vi "readU16.vi"(8 "error in (no error)":errorcluster, 11 "ModbusBuffer in":refnum<class "ModbusBuffer.lvclass">) -> (0 "error out":errorcluster, 2 "Output":u16, 3 "ModbusBuffer out":refnum<class "ModbusBuffer.lvclass">)   [LabVIEW 2016, in "RTModbus.lvlib" / "ModbusBuffer.lvclass"]
uses:
  ModbusBuffer.lvclass
  ModbusBuffer.lvclass/ModbusBuffer.ctl
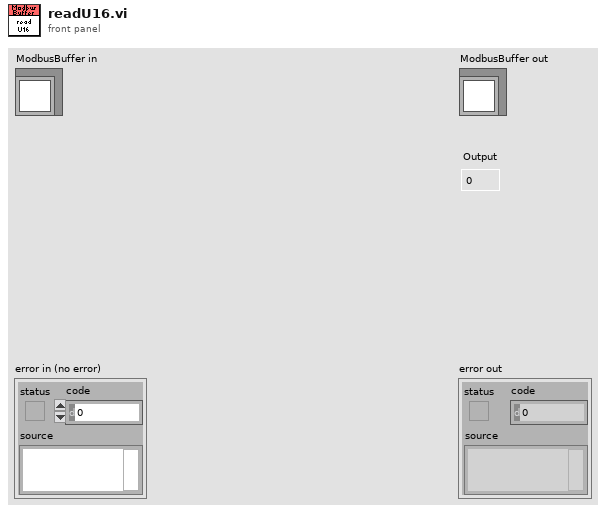
[diagram p1: front panel]
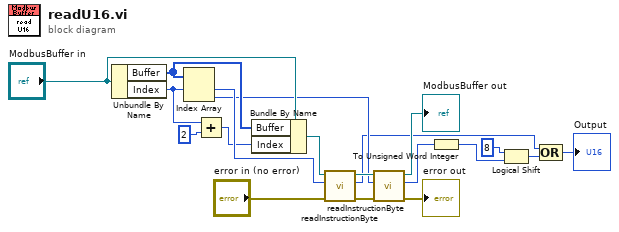
[diagram p0: block diagram]
diagram:
  n1 = Unbundle By Name("ModbusBuffer in") -> ("Buffer"=w18:u16[], "Index"=w14:i32)
  n2 = Index Array(array=w18, index #1=w14) -> (element #1=w17:u16, element #2=w9:u16)  [unwired: 1 in]
  n3 = Add(x=w14, y=2) -> (x+y=w12:i32)
  n4 = Bundle By Name(cluster="ModbusBuffer in", "Buffer"=w18, "Index"=w12) -> (w16:refnum<class "ModbusBuffer.lvclass">)
  n5 = call "readInstructionByte.vi"("error in (no error)"="error in (no error)", "Instruction"=w17, "ModbusBuffer in"=w16) -> ("error out"=w7:errorcluster, "Output"=w8:u8, "ModbusBuffer out"=w11:refnum<class "ModbusBuffer.lvclass">)  [unwired: 6 in]
  n6 = call "readInstructionByte.vi"("error in (no error)"=w7, "Instruction"=w9, "ModbusBuffer in"=w11) -> ("error out"=→"error out":errorcluster, "Output"=w5:u8, "ModbusBuffer out"=→"ModbusBuffer out":refnum<class "ModbusBuffer.lvclass">)  [unwired: 6 in]
  n7 = To Unsigned Word Integer(number=w5) -> (unsigned 16bit integer=w4:u16)
  n8 = Logical Shift(y=i16 8, x=w4) -> (x << y=w2:u16)
  n9 = Compound Arithmetic op=OR(w8, w2) -> (→"Output":u16)
